vi "parameters table ROI.vi"(8 "error in":errorcluster, 11 "data ROIs":T1) -> (0 "error out":errorcluster, 2 "ROIs Values Data":dbl[][](array[numeric]), 3 "ROIs Values":string[][](table))   [LabVIEW 2023]
uses:
  control/rois list cluster.ctl
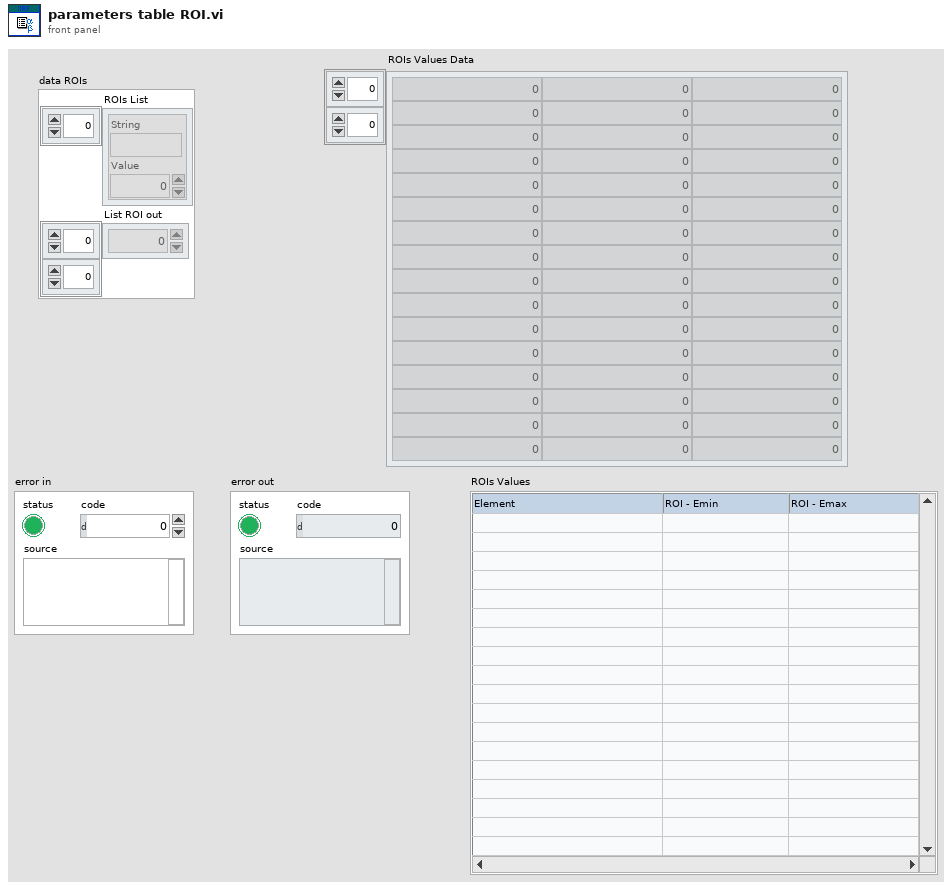
[diagram p1: front panel]
types:
  T1 = typedef "rois list cluster.ctl" = cluster{"ROIs List":cluster{"String":string, "Value":i32}[], "List ROI out":dbl[][]}
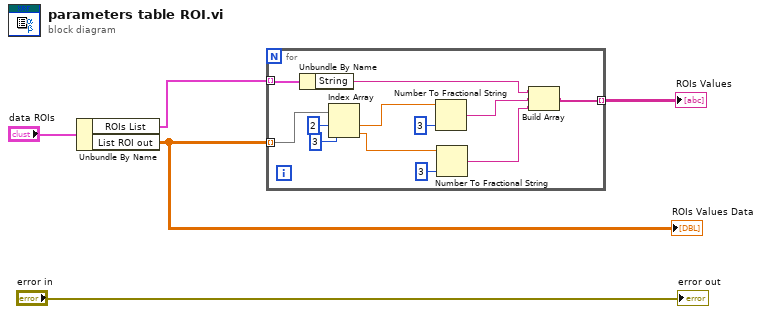
[diagram p0: block diagram]
diagram:
  n1 = Unbundle By Name("data ROIs") -> ("ROIs List"=w4:cluster{"String":string, "Value":i32}[], "List ROI out"=w3:dbl[][])
  "ROIs Values Data" <- w3
  n2 = for {
    tunnel: w4 -> [w17] mode=indexing
    tunnel: w3 -> [w16] mode=indexing
    tunnel: [w6] -> w1 mode=indexing
    n3 = Unbundle By Name(w17) -> ("String"=w7:string)
    n4 = Index Array(array=w16, index #1=2 ("index"), index #2=3 ("index")) -> (element #1=w13:dbl, element #2=w10:dbl)
    n5 = Number To Fractional String(number=w13, precision (6)=i16 3) -> (F-format string=w8:string)  [unwired: 2 in]
    n6 = Number To Fractional String(number=w10, precision (6)=i16 3) -> (F-format string=w9:string)  [unwired: 2 in]
    n7 = Build Array(w7, w8, w9) -> (w6:string[])
  }
  "ROIs Values" <- w1
  "error out" <- "error in"
